vi "test external trigger.vi"() -> ()   [LabVIEW 2017]
uses:
  <vilib>/DAQmx/read.llb/DAQmx Read (Analog 1D DBL 1Chan NSamp).vi
  <vilib>/DAQmx/create/channels.llb/DAQmx Create Channel (AI-Voltage-Basic).vi
  <vilib>/DAQmx/configure/timing.llb/DAQmx Timing (Sample Clock).vi
  <vilib>/DAQmx/miscellaneous.llb/DAQmx Fill In Error Info.vi
  <vilib>/Analysis/NI_AALBase.lvlib
panel:
  out "output array":dbl[](array[numeric])
  out "error out":errorcluster
  in  "Points per loop":i32=50
  in  "Trigger source":tag="/Dev1/APFI0"
  in  "Sample Rate":dbl=50.0 format="%.3p"
  in  "Voltage Read":tag="Dev1/ai1"
  in  "Points Number":i32=1000
  in  "intervals":i32=100
  out "Histogram Graph":T1(graph)={"X Values"=[1.3335459541621144, 1.3348573631903649, 1.3361687722186153, 1.3374801812468657, 1.3387915902751162, 1.3401029993033666, 1.341414408331617, 1.3427258173598675, 1.344037226388118, 1.3453486354163684, 1.3466600444446188, 1.3479714534728693, 1.3492828625011197, 1.3505942715293702, 1.3519056805576206, 1.353217089585871, 1.3545284986141215, 1.355839907642372, 1.3571513166706224, 1.3584627256988728, 1.3597741347271233, 1.3610855437553737, 1.3623969527836242, 1.3637083618118746, 1.365019770840125, 1.3663311798683755, 1.367642588896626, 1.3689539979248764, 1.3702654069531268, 1.3715768159813773, 1.3728882250096277, 1.3741996340378781, 1.3755110430661286, 1.376822452094379, 1.3781338611226295, 1.37944527015088, 1.3807566791791304, 1.3820680882073808, 1.3833794972356313, 1.3846909062638817, 1.3860023152921321, 1.3873137243203826, 1.388625133348633, 1.3899365423768835, 1.391247951405134, 1.3925593604333844, 1.3938707694616348, 1.3951821784898852, 1.3964935875181357, 1.3978049965463861, 1.3991164055746366, 1.400427814602887, 1.4017392236311375, 1.403050632659388, 1.4043620416876383, 1.4056734507158888, 1.4069848597441392, 1.4082962687723897, 1.4096076778006401, 1.4109190868288906, 1.412230495857141, 1.4135419048853914, 1.4148533139136419, 1.4161647229418923, 1.4174761319701428, 1.4187875409983932, 1.4200989500266437, 1.421410359054894, 1.4227217680831445, 1.424033177111395, 1.4253445861396454, 1.4266559951678959, 1.4279674041961463, 1.4292788132243968, 1.4305902222526472, 1.4319016312808976, 1.433213040309148, 1.4345244493373985, 1.435835858365649, 1.4371472673938994, 1.4384586764221499, 1.4397700854504003, 1.4410814944786507, 1.4423929035069012, 1.4437043125351516, 1.445015721563402, 1.4463271305916525, 1.447638539619903, 1.4489499486481534, 1.4502613576764039, 1.4515727667046543, 1.4528841757329047, 1.4541955847611552, 1.4555069937894056, 1.456818402817656, 1.4581298118459065, 1.459441220874157, 1.4607526299024074, 1.4620640389306578, 1.4633754479589083], "Histogram: h(x)"=[1, 0, 0, 0, 0, 0, 0, 0, 0, 0, 0, 0, 0, 0, 0, 0, 0, 0, 0, 0, 0, 0, 0, 0, 0, 0, 0, 0, 0, 0, 0, 0, 0, 0, 0, 0, 0, 0, 0, 0, 0, 0, 0, 0, 0, 0, 0, 0, 0, 0, 0, 0, 1, 2, 0, 0, 0, 0, 1, 2, 2, 2, 4, 4, 10, 12, 8, 14, 19, 15, 27, 41, 56, 77, 73, 95, 133, 147, 191, 208, 218, 275, 292, 337, 357, 423, 345, 321, 302, 262, 210, 181, 176, 61, 38, 29, 13, 5, 7, 3]}
  in  "stop":bool
  out "Points get":i32=5000
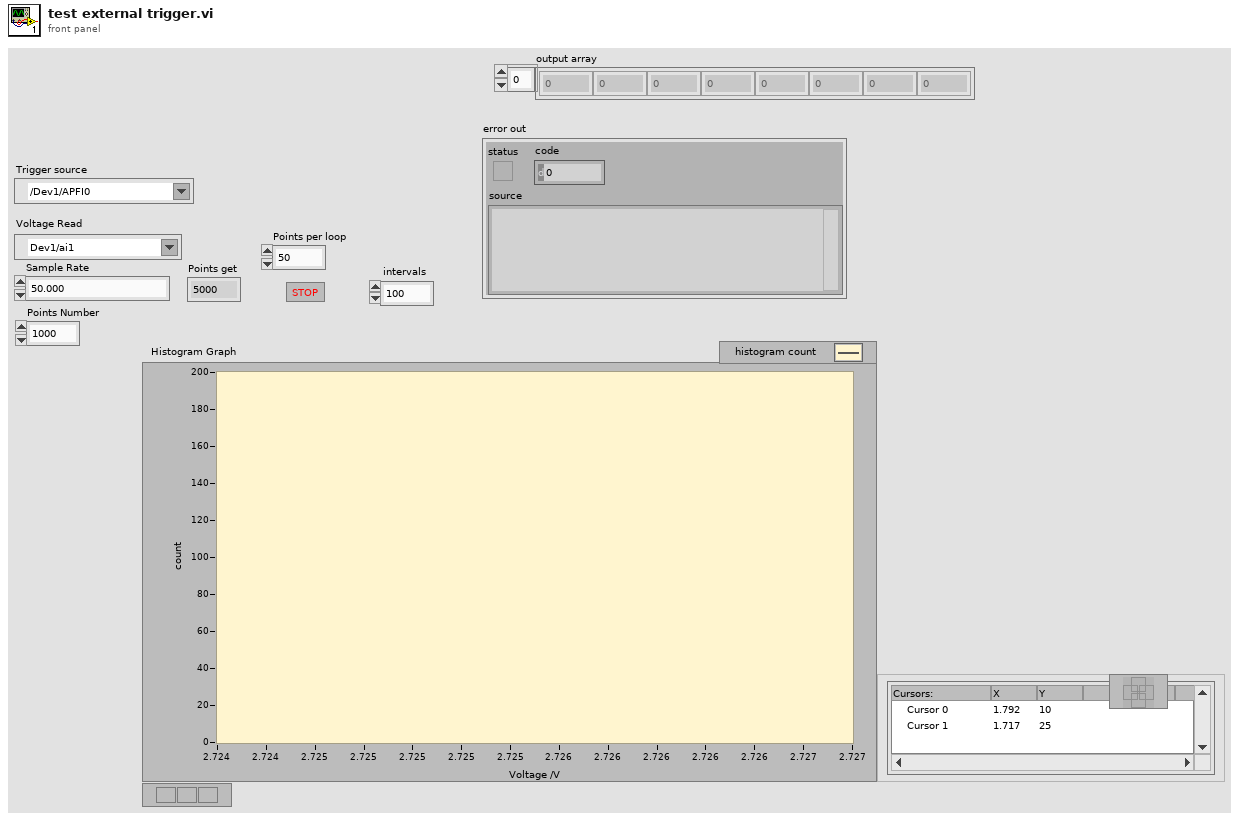
[diagram p1: front panel]
types:
  T1 = cluster{"X Values":dbl[], "Histogram: h(x)":i32[]}
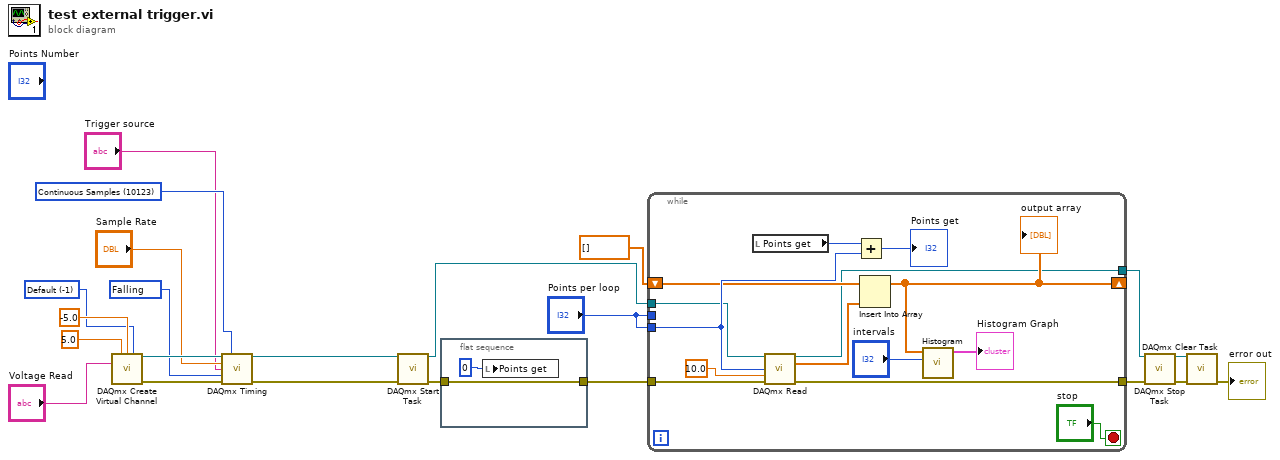
[diagram p0: block diagram]
diagram:
  w14 = 10171 items=["Rising"=10280, "Falling"=10171] ("active edge")
  w15 = 10123 items=["Finite Samples"=10178, "Continuous Samples"=10123, "Hardware Timed Single Point"=12522] ("sample mode")
  w18 = -1 items=["Default"=-1, "RSE"=10083, "NRSE"=10078, "Differential"=10106, "Pseudodifferential"=12529] ("input terminal configuration")
  n1 = call-poly <vilib>:"DAQmx Create Virtual Channel.vi"("maximum value"=5.0, "minimum value"=-5.0, "input terminal configuration"=w18, "physical channels"="Voltage Read") -> ("task out"=w17:refnum<k21>, "error out"=w6:errorcluster)  [unwired: 10 in]
  n2 = call-poly <vilib>:"DAQmx Timing.vi"("task/channels in"=w17, "sample mode"=w15, "rate"="Sample Rate", "source"="Trigger source", "active edge"=w14, "error in"=w6) -> ("task out"=w2:refnum<k21>, "error out"=w13:errorcluster)  [unwired: 8 in]
  n3 = call <vilib>:"DAQmx Start Task.vi"("task/channels in"=w2, "error in"=w13) -> ("task out"=w12:refnum<k21>, "error out"=w4:errorcluster)  [unwired: 12 in]
  n4 = flat-sequence {
    tunnel: w4 -> [w24]
    tunnel: [w24] -> w3
    frame #0 {
      n5 = local write "Points get"(0 ("Points get")) -> ()
    }
  }
  n6 = while {
    shift-right: [w32] -> _
    shift-left: dbl[] [] -> [w33]
    tunnel: [w31] -> w9
    tunnel: "Points per loop" -> [w34]
    tunnel: w12 -> [w29]
    tunnel: w3 -> [w28]
    tunnel: [w30] -> w8
    tunnel: "Points per loop" -> [_]
    stop <- "stop" stop-if-true
    n7 = local read "Points get"() -> (w27:i32)
    n8 = call-poly <vilib>:"DAQmx Read.vi"("task/channels in"=w29, "number of samples per channel"=w34, "timeout"=10.0, "error in"=w28) -> ("task out"=w30:refnum<k21>, "data"=w25:dbl[], "error out"=w31:errorcluster)  [unwired: 9 in]
    n9 = Add(x=w27, y=w34) -> (x+y=→"Points get":i32)
    n10 = Insert Into Array(array=w33, new element=w25) -> (w32:dbl[])  [unwired: 1 in]
    "output array" <- w32
    n11 = call <vilib>:"Histogram.vi"("intervals"="intervals", "X"=w32) -> ("Histogram Graph"=→"Histogram Graph":T1)  [unwired: 6 in, 3 out]
  }
  n12 = call <vilib>:"DAQmx Stop Task.vi"("task/channels in"=w8, "error in"=w9) -> ("task out"=w11:refnum<k21>, "error out"=w10:errorcluster)  [unwired: 12 in]
  n13 = call <vilib>:"DAQmx Clear Task.vi"("task in"=w11, "error in"=w10) -> ("error out"=→"error out":errorcluster)  [unwired: 13 in]
